vi "PipBoy_Cmd-Previous.vi"(8 "error in (no error)":errorcluster, 11 "DataIn":T1) -> (0 "error out":errorcluster, 3 "DataOut":T1)   [LabVIEW 2014]
uses:
  ctls/PipBoy_PipBoyData.ctl
  ctls/PipBoy_ProcComm.ctl
  System.Windows.Forms
  ctls/PipBoy_PipBoyCommand.ctl
  ctls/PipBoy_Message.ctl
  modules/support/Message Queue/All Message Queues.ctl
  modules/support/Message Queue/Message Cluster.ctl
  ctls/PipBoy_FileConf.ctl
  ctls/PipBoy_PicComm.ctl
  ctls/PipBoy_GeneralParams.ctl
  ctls/PipBoy_Pages.ctl
  modules/support/Message Queue/Message Queue.lvlib
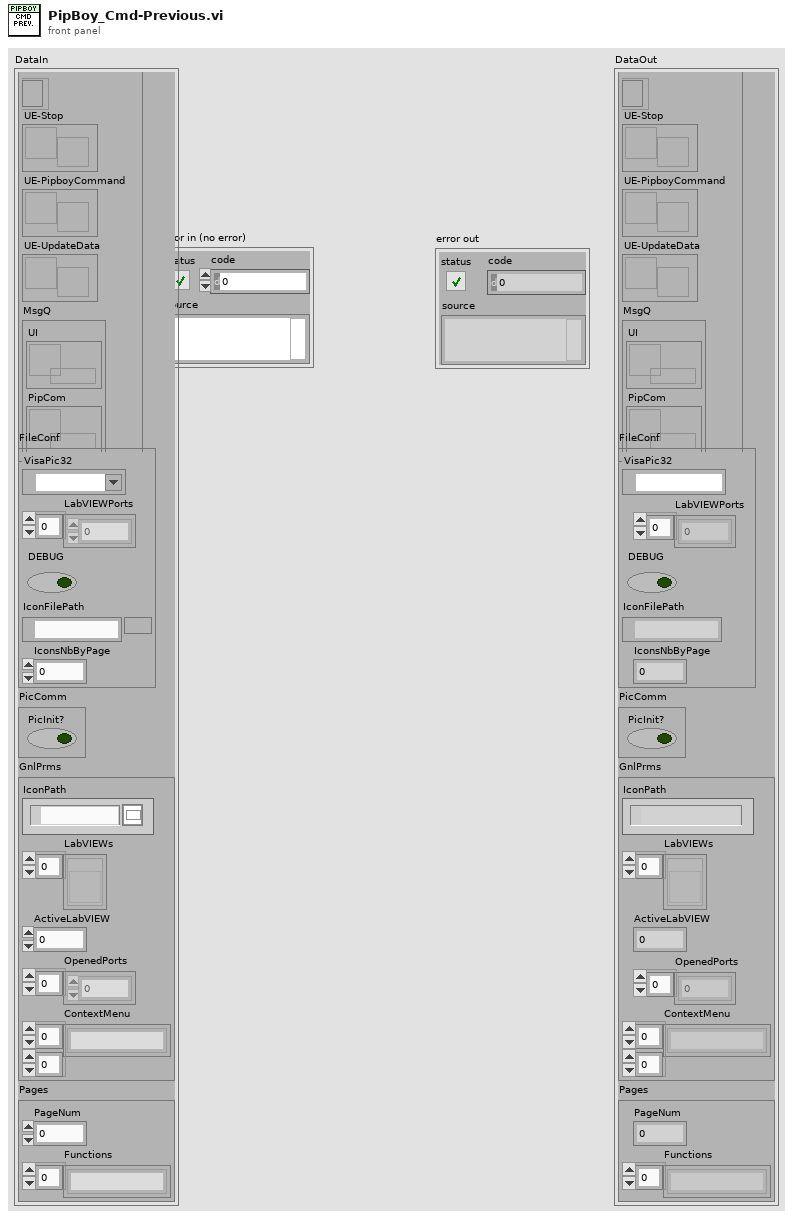
[diagram p1: front panel]
types:
  T1 = typedef "PipBoy_PipBoyData.ctl" = cluster{"ProcComm":T2, "FileConf":T4, "PicComm":T5, "GnlPrms":T6, "Pages":T7}
  T2 = typedef "PipBoy_ProcComm.ctl" = cluster{"NotifyIconRef":refnum<k24>, "UE-Stop":refnum<user-event>, "UE-PipboyCommand":refnum<user-event>, "UE-UpdateData":refnum<user-event>, "MsgQ":T3}
  T3 = typedef "Message Queue.lvlib/All Message Queues.ctl" = cluster{"UI":refnum<queue>, "PipCom":refnum<queue>}
  T4 = typedef "PipBoy_FileConf.ctl" = cluster{"VisaPic32":refnum<visa-resource-name>, "LabVIEWPorts":u16[], "DEBUG":bool, "IconFilePath":path, "IconsNbByPage":i32}
  T5 = typedef "PipBoy_PicComm.ctl" = cluster{"PicInit?":bool}
  T6 = typedef "PipBoy_GeneralParams.ctl" = cluster{"IconPath":path, "LabVIEWs":refnum<vi>[], "ActiveLabVIEW":i32, "OpenedPorts":u16[], "ContextMenu":string[][]}
  T7 = typedef "PipBoy_Pages.ctl" = cluster{"PageNum":i32, "Functions":string[]}
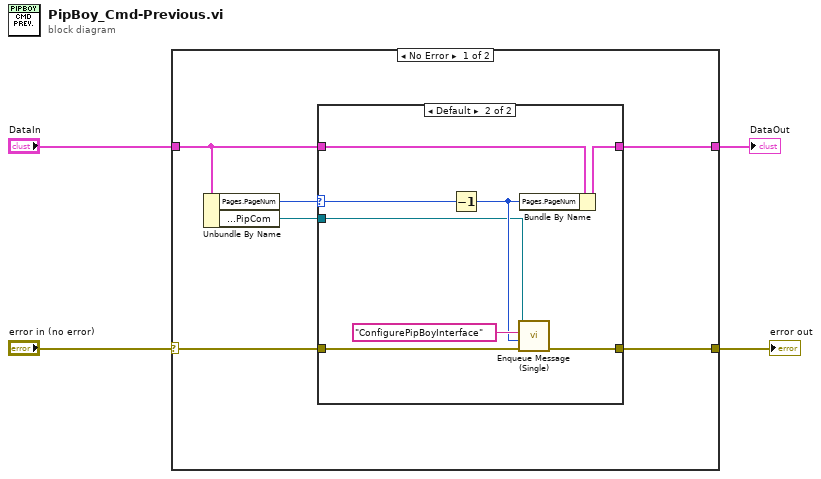
[diagram p0: block diagram]
diagram:
  n1 = case shown="No Error" "error in (no error)" {
    selector: "error in (no error)" -> [w9 w22]
    tunnel: [w8 w22] -> w4
    tunnel: "DataIn" -> [w7 w21]
    tunnel: [w6 w21] -> w1
    frame No Error {
      n2 = Unbundle By Name(w7) -> ("Pages.PageNum"=w5:i32, "ProcComm.MsgQ.PipCom"=w10:refnum<queue>)
      n3 = case shown="Default" w5 {
        selector: w5 -> [_ w15]
        tunnel: w10 -> [_ w18]
        tunnel: w9 -> [w12 w17]
        tunnel: [w12 w16] -> w8
        tunnel: w7 -> [w11 w14]
        tunnel: [w11 w13] -> w6
        frame 0 {
        }
        frame Default {
          n4 = Decrement(x=w15) -> (x-1=w19:i32)
          n5 = call "Enqueue Message (Single).vi"("error in (no error)"=w17, "Message Data"=w19, "Message"="ConfigurePipBoyInterface", "Message Queue"=w18) -> ("error out"=w16:errorcluster)  [unwired: 6 in, 1 out]
          n6 = Bundle By Name(cluster=w14, "Pages.PageNum"=w19) -> (w13:T1)
        }
      }
    }
    frame Error {
    }
  }
  "error out" <- w4
  "DataOut" <- w1
